vi "LogFFT with2xpadding.vi"(5 "FFT Pad?":bool, 9 "Padded FT Size":i32, 10 "FFT {X}":cdb[](array[numeric])) -> (2 "Log{Mag(FFT)}":dbl[](array[numeric]))   [LabVIEW 2012]
uses:
  <vilib>/Analysis/2dsp.llb/Inverse Complex FFT.vi
  <vilib>/Analysis/NI_AALPro.lvlib
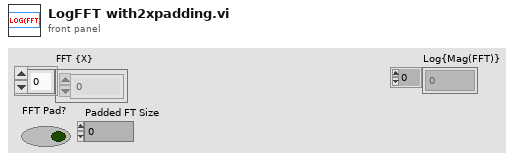
[diagram p1: front panel]
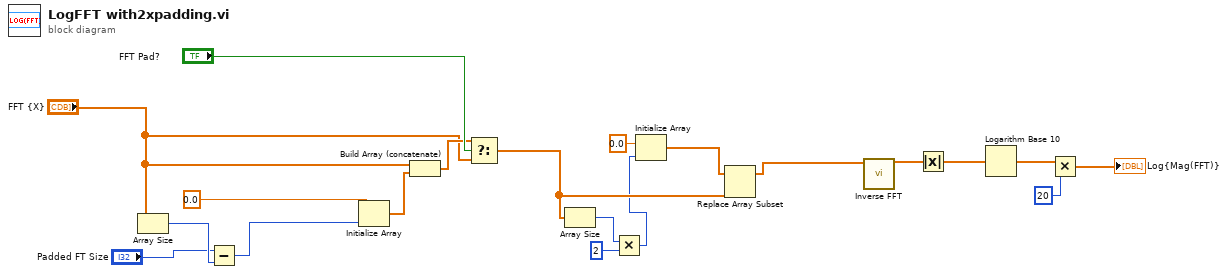
[diagram p0: block diagram]
diagram:
  n1 = Array Size(array="FFT {X}") -> (size(s)=w12:i32)
  n2 = Subtract(x="Padded FT Size", y=w12) -> (x-y=w10:i32)
  n3 = Initialize Array(0.0 ("element"), w10) -> (w15:dbl[])
  n4 = Build Array (concatenate)("FFT {X}", w15) -> (w13:cdb[])
  n5 = Select(t=w13, s="FFT Pad?", f="FFT {X}") -> (s? t:f=w5:cdb[])
  n6 = Array Size(array=w5) -> (size(s)=w3:i32)
  n7 = Multiply(x=w3, y=2) -> (x*y=w2:i32)
  n8 = Initialize Array(0.0 ("element"), w2) -> (w6:dbl[])
  n9 = Replace Array Subset(array=w6, new element=w5) -> (w4:dbl[])  [unwired: 1 in]
  n10 = call-poly <vilib>:"Inverse FFT.vi"("FFT {X}"=w4) -> ("X"=w9:cdb[])  [unwired: 9 in, 1 out]
  n11 = Absolute Value(x=w9) -> (abs(x)=w17:dbl[])
  n12 = Logarithm Base 10(1:w17) -> (0:w20:dbl[])
  n13 = Multiply(x=w20, y=20) -> (x*y=→"Log{Mag(FFT)}":dbl[])
